vi "COVIDxPLORE.vi"() -> ()   [LabVIEW 2017]
panel:
  in  "LeftTab":enum32{"Page 1", "Page 2"}(tab)
  out "How many days until zero growth?":string
  out "Is there a trend in the growth?":string
  out "Is the infection growing?":string
  out "What part of the population is infected?":string
  out "How many are infected?":string
  out "How many days until zero growth?":string
  out "Is there a trend in the growth of dead?":string
  out "Are the number of dead growing?":string
  out "What part of the population has died?":string
  out "How many are dead?":string
  in  "RightTabs":enum32{"Plots", "GeoSelect"}(tab)
  in  "Fixed":T1
  in  "Days":i32
  in  "ZoomToDays":bool
  in  "ResetGraph":bool
  in  "GotoGeo":bool
  in  "Plots":u16(ring) items=["Modoc County Dead", "Modoc County Infected", "Siskiyou County Dead", "Siskiyou County Infected", "Humboldt County Dead", "Humboldt County Infected", "Washoe County Dead", "Washoe County Infected", "Benton County Dead", "Benton County Infected", "Crook County Dead", "Crook County Infected", "Deschutes County Dead", "Deschutes County Infected", "Douglas County Dead", "Douglas County Infected", "Grant County Dead", "Grant County Infected", "Harney County Dead", "Harney County Infected", "Jackson County Dead", "Jackson County Infected", "Jefferson County Dead", "Jefferson County Infected", "Klamath County Dead", "Klamath County Infected", "Lake County Dead", "Lake County Infected", "Lane County Dead", "Lane County Infected", "Lincoln County Dead", "Lincoln County Infected", "Linn County Dead", "Linn County Infected", "Marion County Dead", "Marion County Infected", "Wasco County Dead", "Wasco County Infected", "Combined Dead", "Combined Infected"]
  out "Plot":cluster{"Days":timestamp[], dbl[]}[](graph)
  in  "GotoPlots":bool
  in  "Clear":bool
  in  "Level":u16(ring) items=["County", "State", "Country"]
  in  "Expand":bool
  in  "Add":bool
  out "Days of data":i32
  out "Last day of data":timestamp format="%<%m/%d>T"
  out "Regions":string[][](table)
  in  "Lookup":bool
  in  "Find by":u16(ring) items=["Zipcode", "CountyName", "StateName", "CountyFips", "StateFips", "StateAbbr", "CityState"]
  in  "GeoData":T2
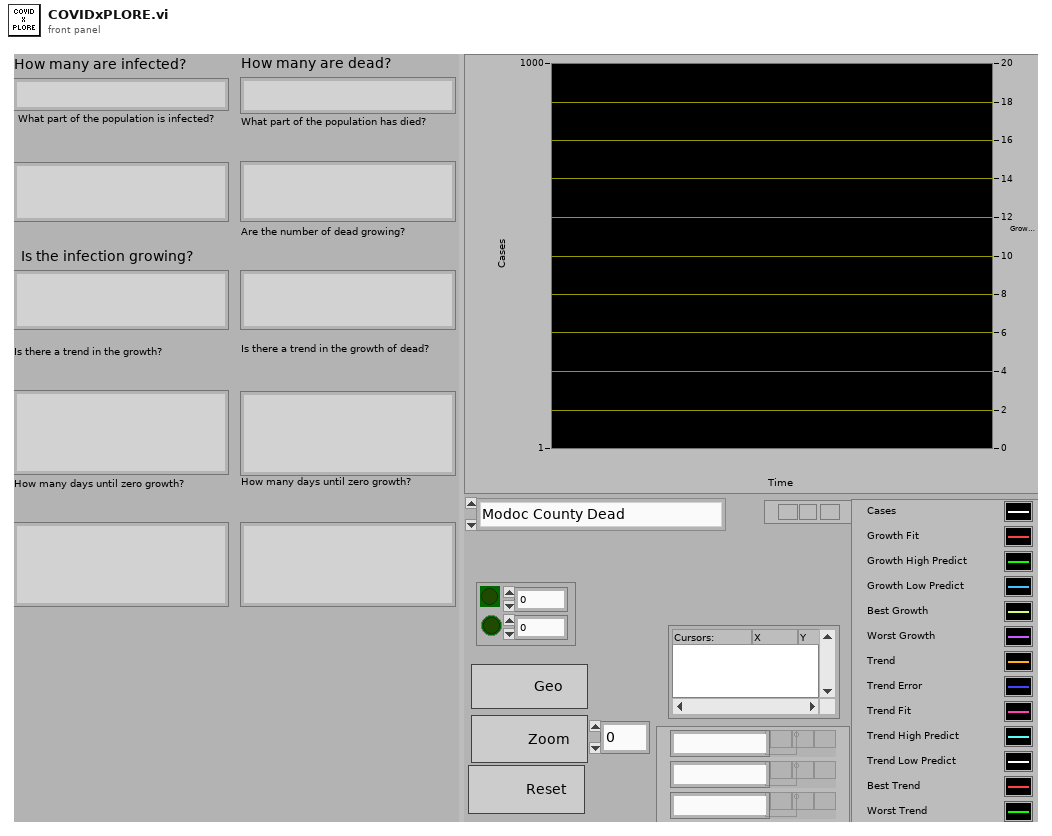
[diagram p1: front panel]
types:
  T1 = cluster{"FixedGrowth":bool, "DaysBackGrowth":dbl, "FixedTrend":bool, "DaysBackTrend":dbl}
  T2 = cluster{"Zip":i32, "CountyFIPS":i32, "StateFips":i32, "CountyName":string, "StateName":string, "StateAbbr":string, "City":string}
  T3 = enum16{"LoadData", "GetStateData", "GetCountyData", "GetCountyArray"}
  T4 = enum16{"ClearCache", "AddPlot", "GetPlot", "GetNames", "LastPlot"}
  T5 = enum16{"Zipcode", "CountyName", "StateName", "CountyFips", "StateFips", "StateAbbr", "CityState"}
  T6 = enum16{"AddEntry", "Clear", "Expand", "Combine", "GetStrings"}
  T7 = enum16{"AddEntry", "Clear", "Expand", "Combine", "GetStrings", "GetGeo"}
  T8 = cluster{"Infected":string, "InfectedRate":string, "InfectionGrowth":string, "GrowthTrend":string, "DaysToZero":string, "Dead":string, "CFR":string, "CFR Growth":string, "CFRtrend":string, "DaysToZeroDead":string}
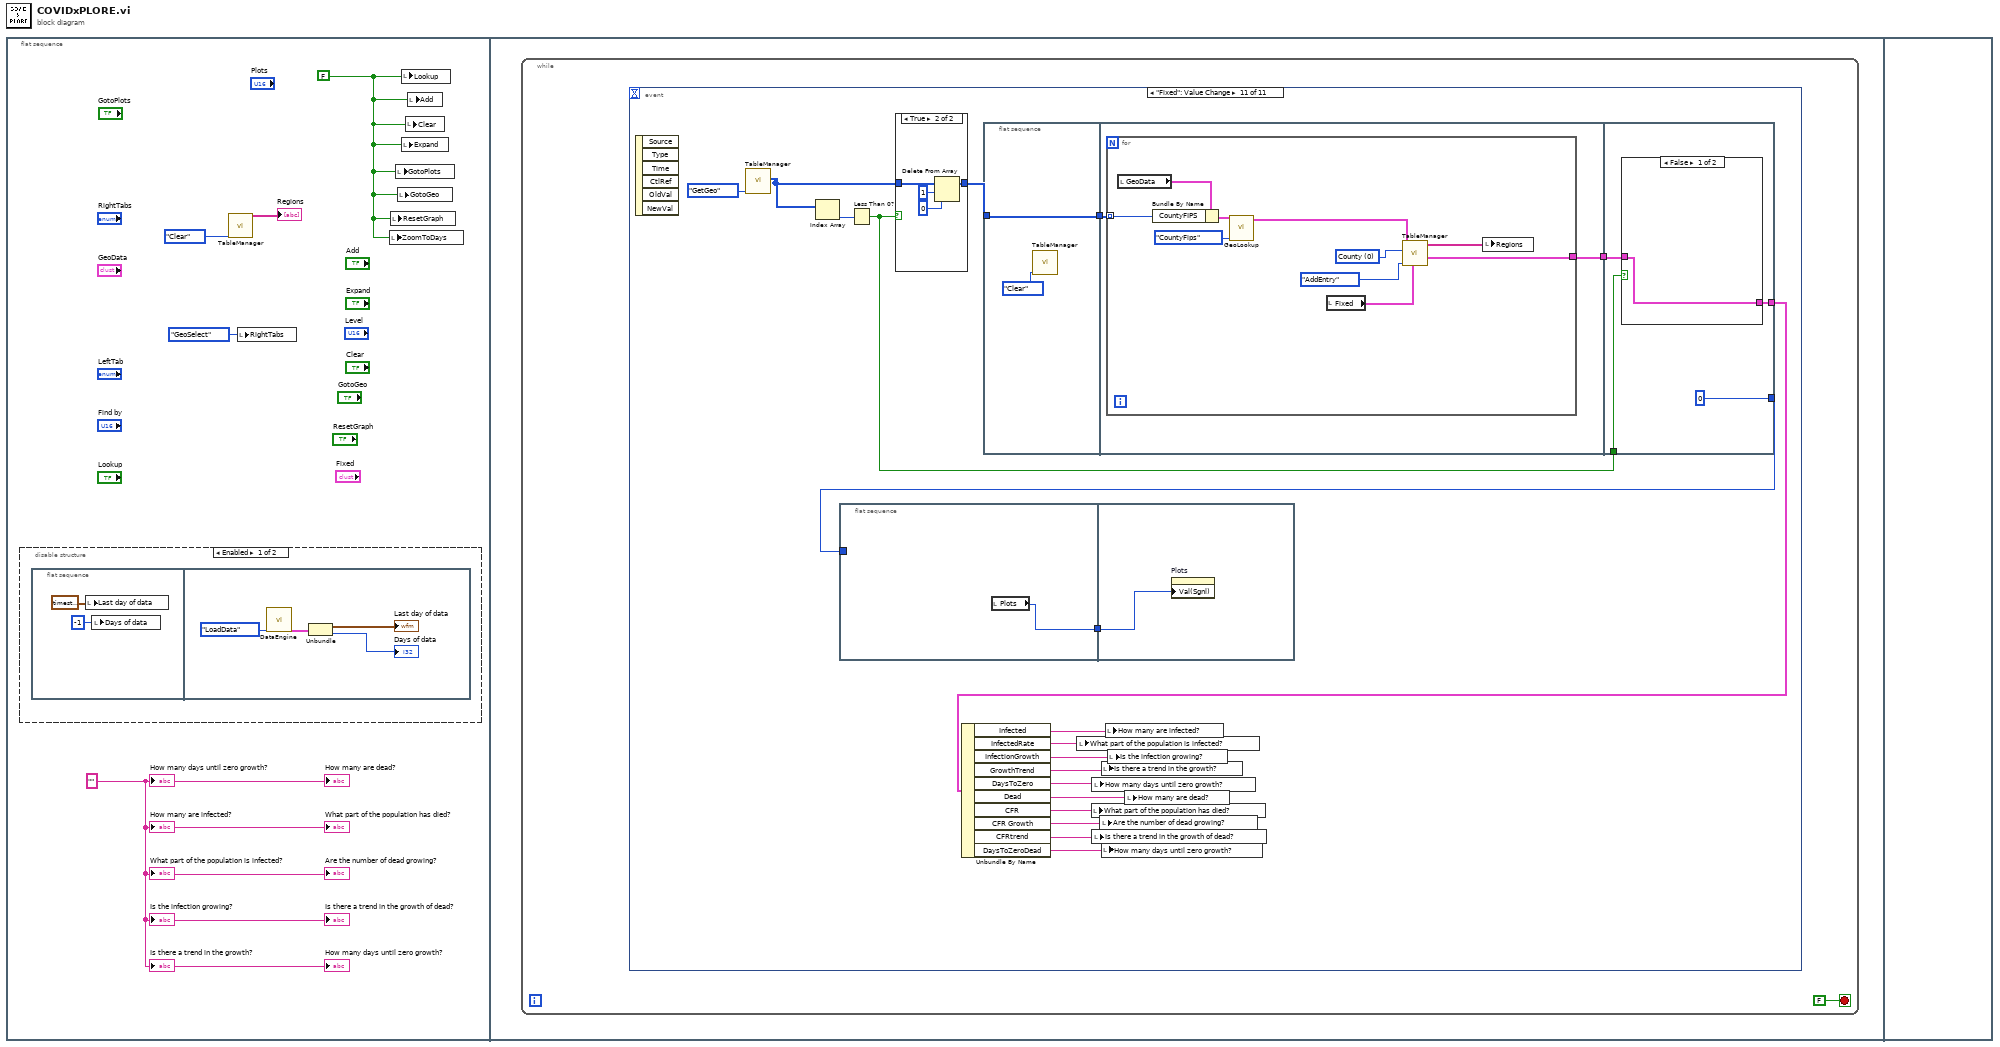
[diagram p0: block diagram]
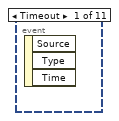
[diagram p3: hidden frame]
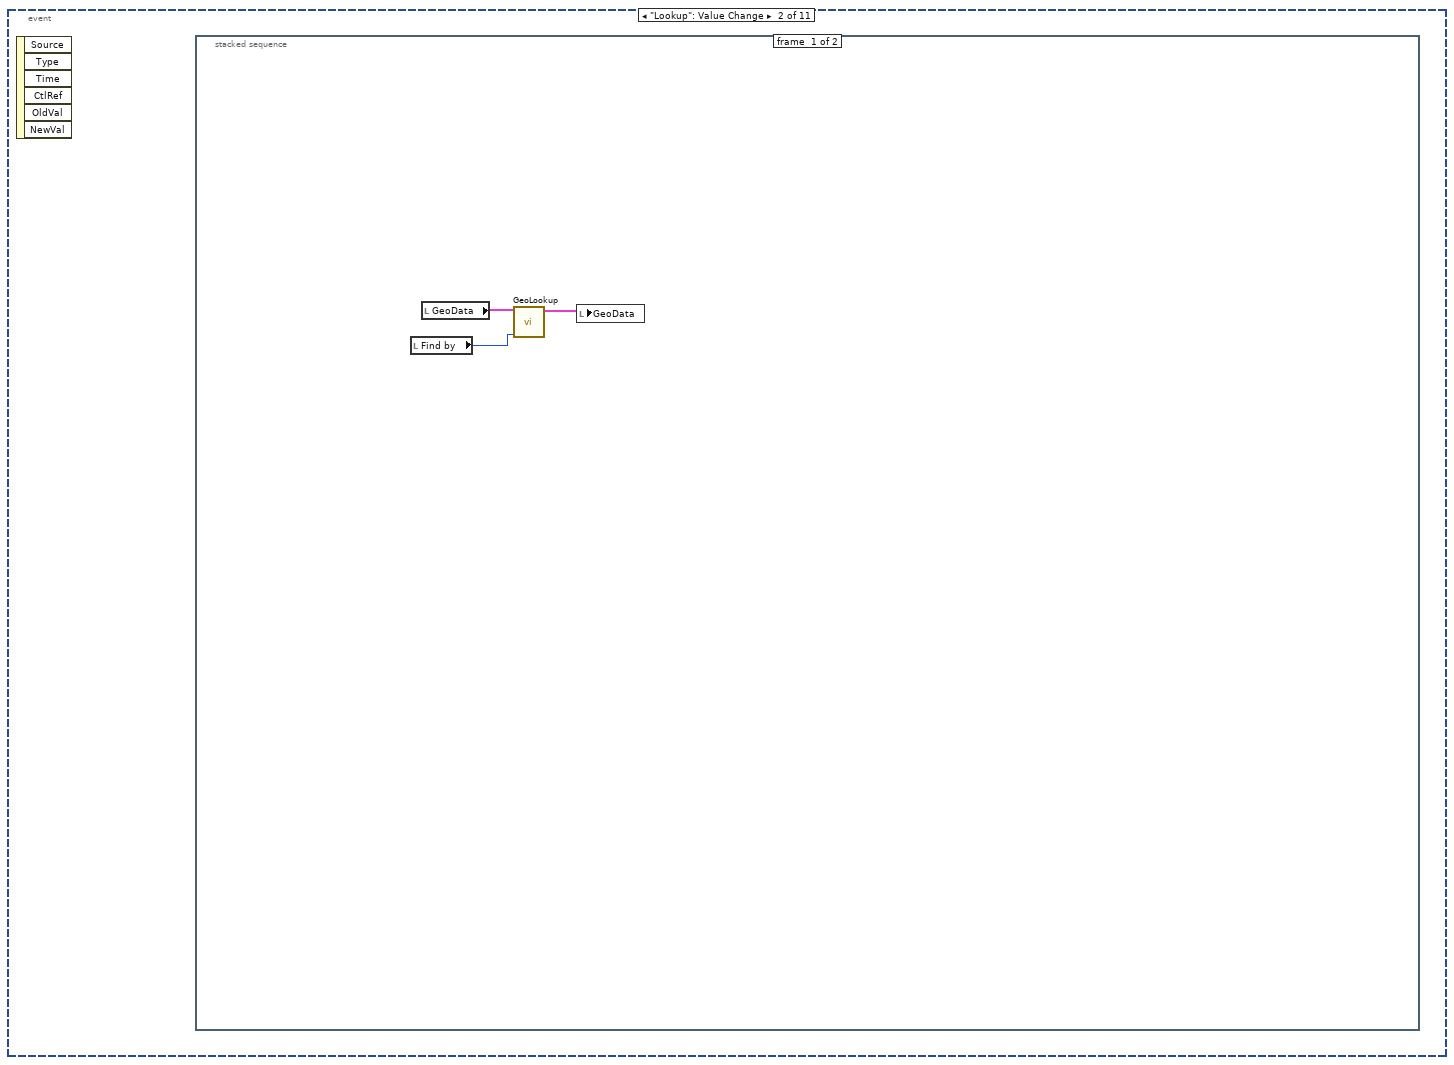
[diagram p4: hidden frame]
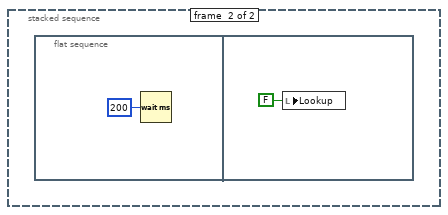
[diagram p5: hidden frame]
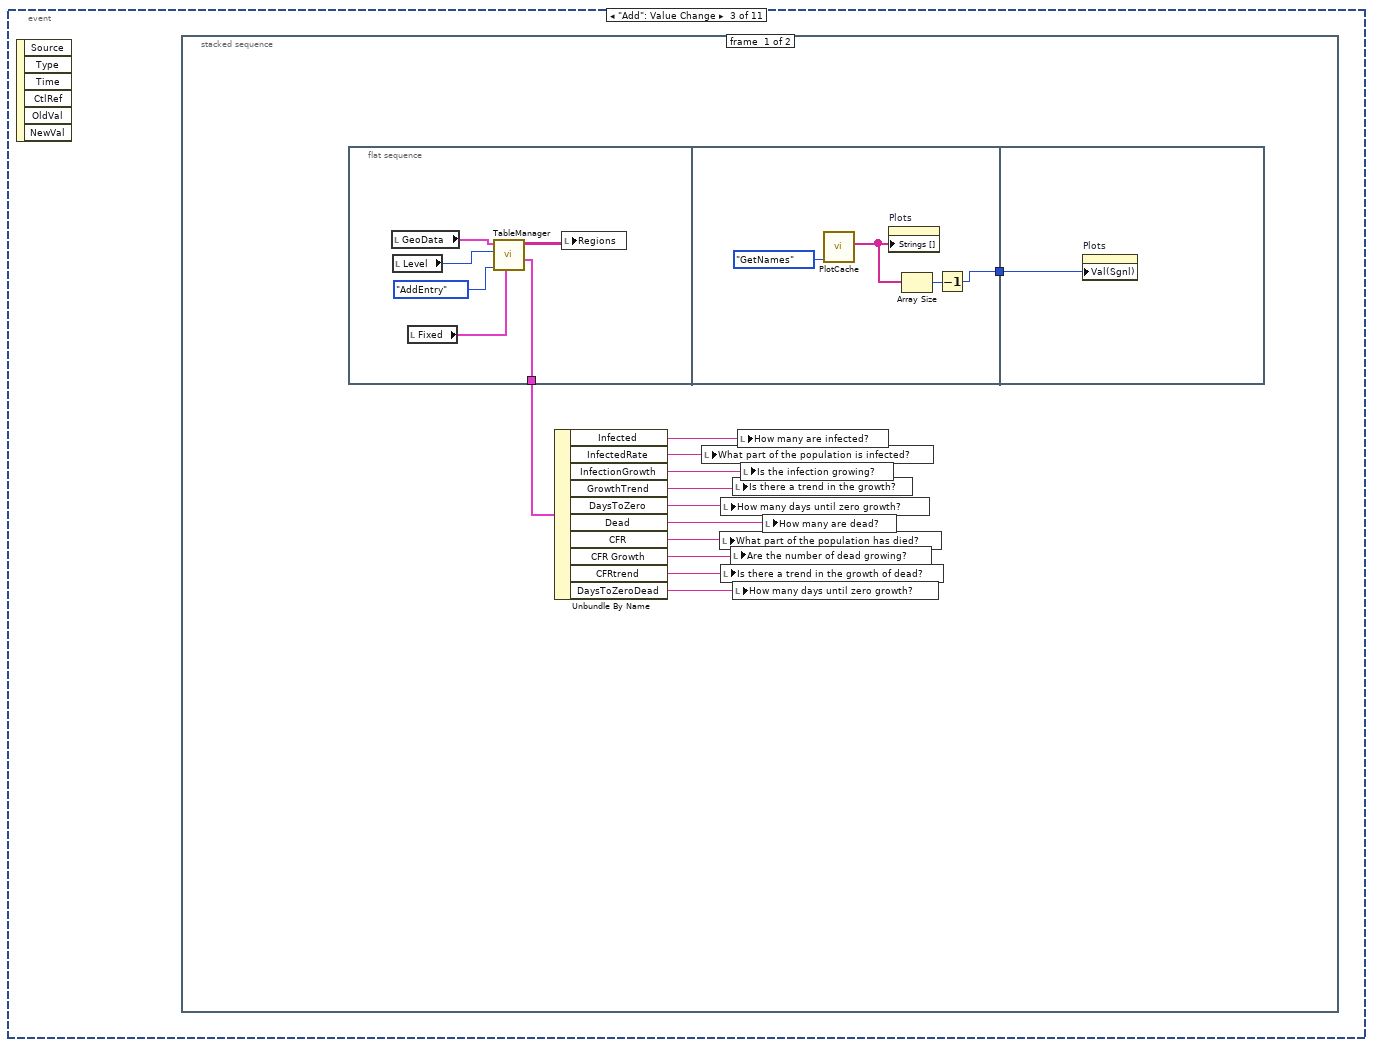
[diagram p6: hidden frame]
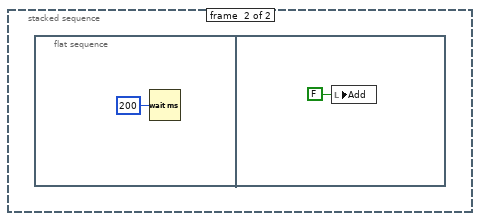
[diagram p7: hidden frame]
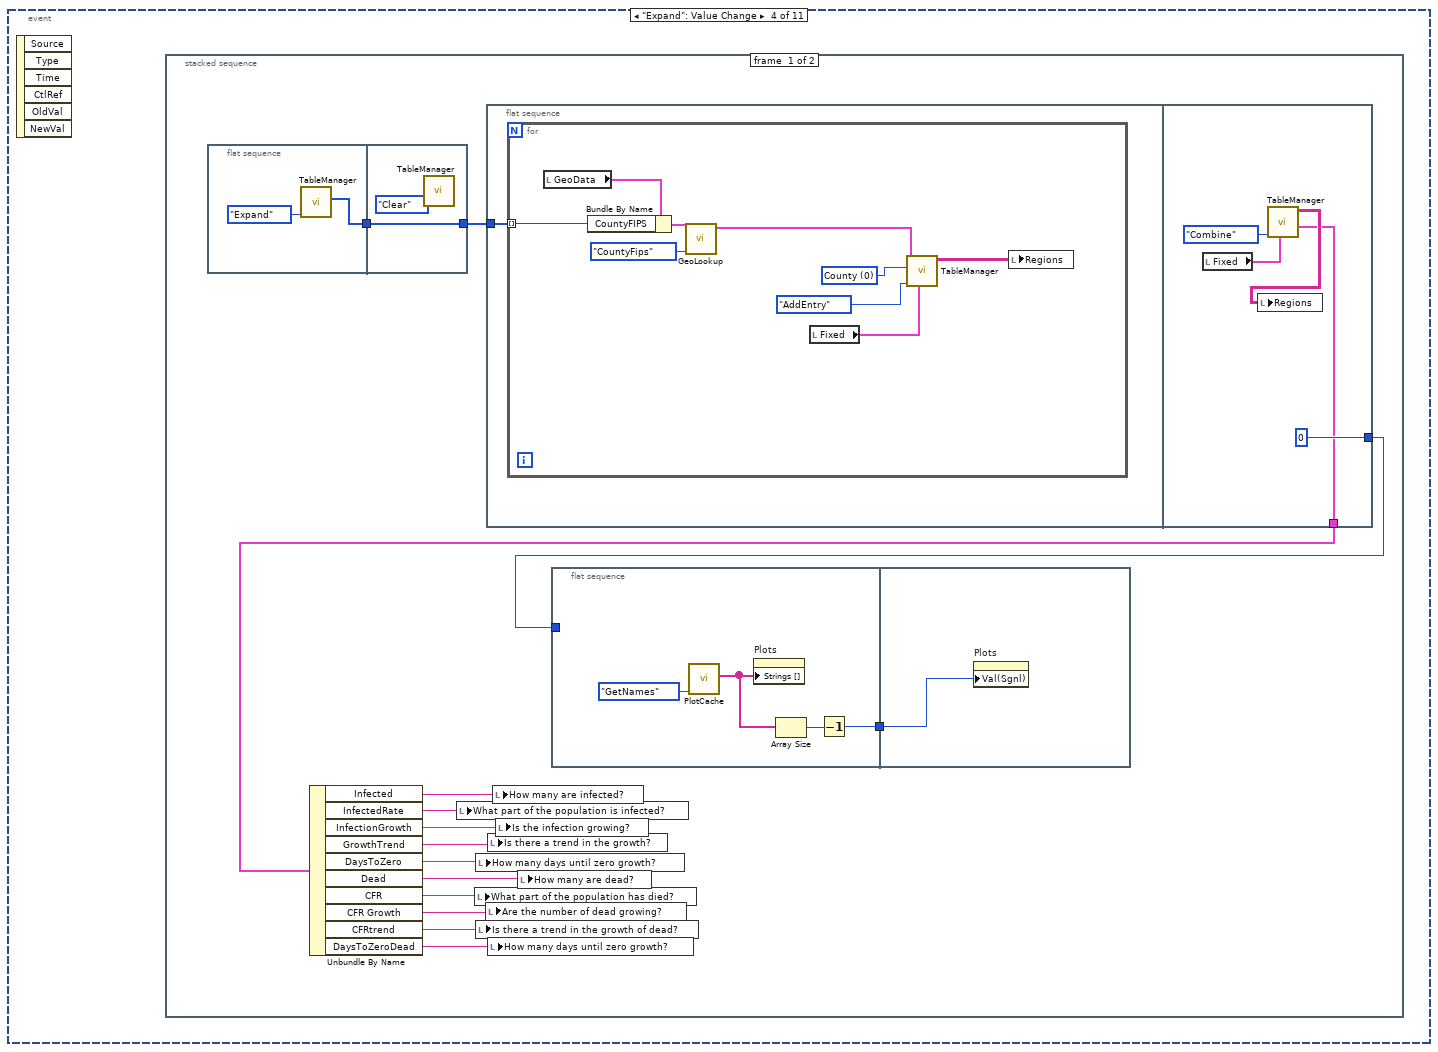
[diagram p8: hidden frame]
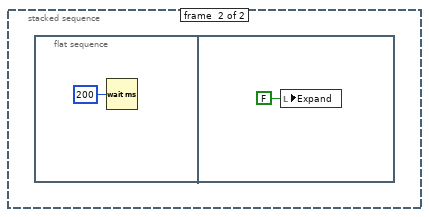
[diagram p9: hidden frame]
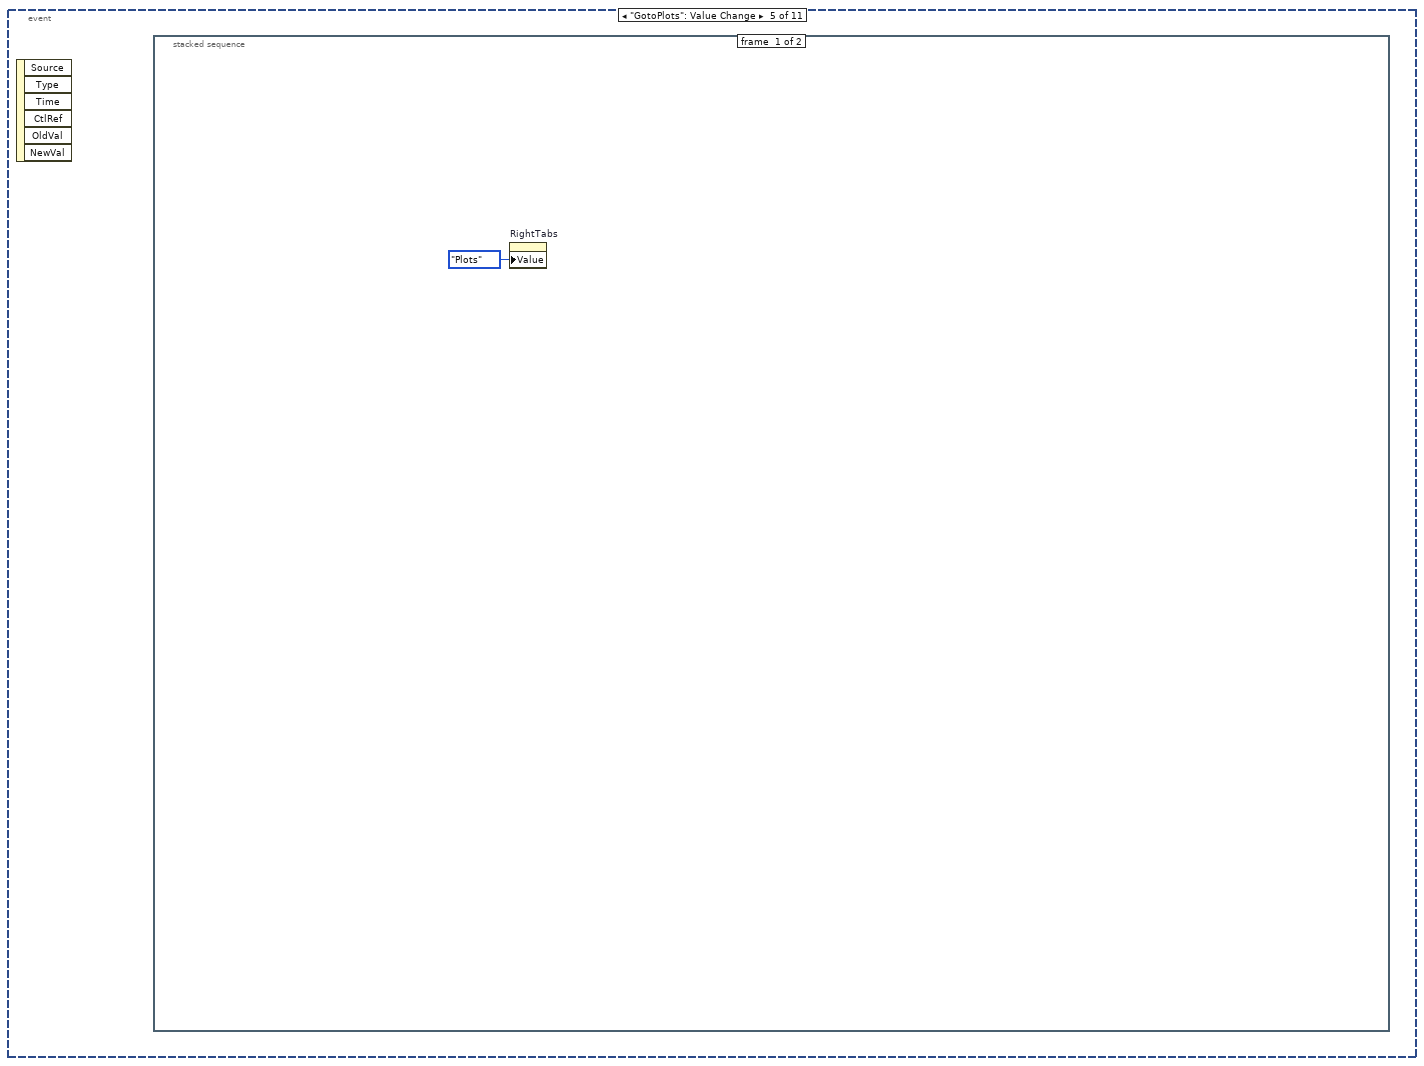
[diagram p10: hidden frame]
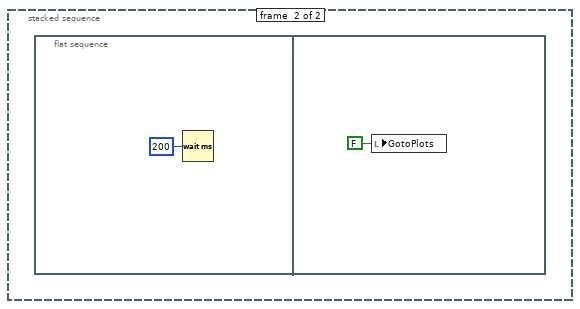
[diagram p11: hidden frame]
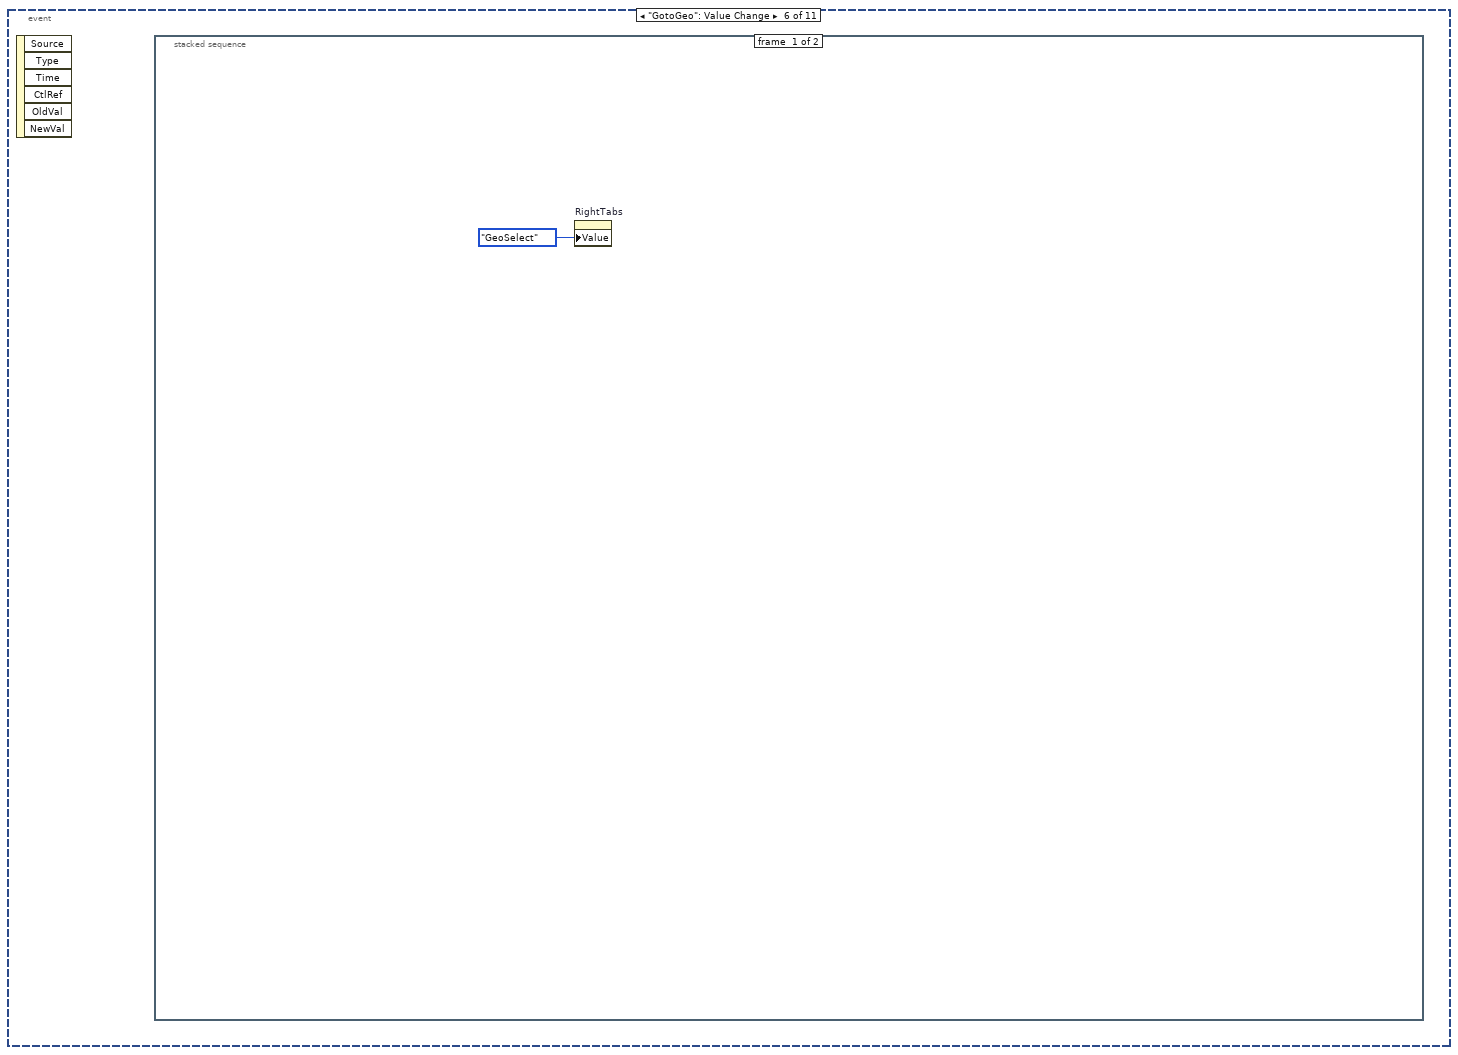
[diagram p12: hidden frame]
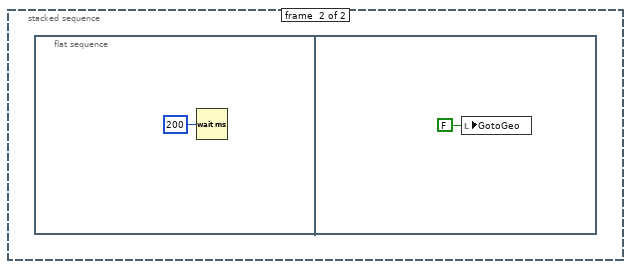
[diagram p13: hidden frame]
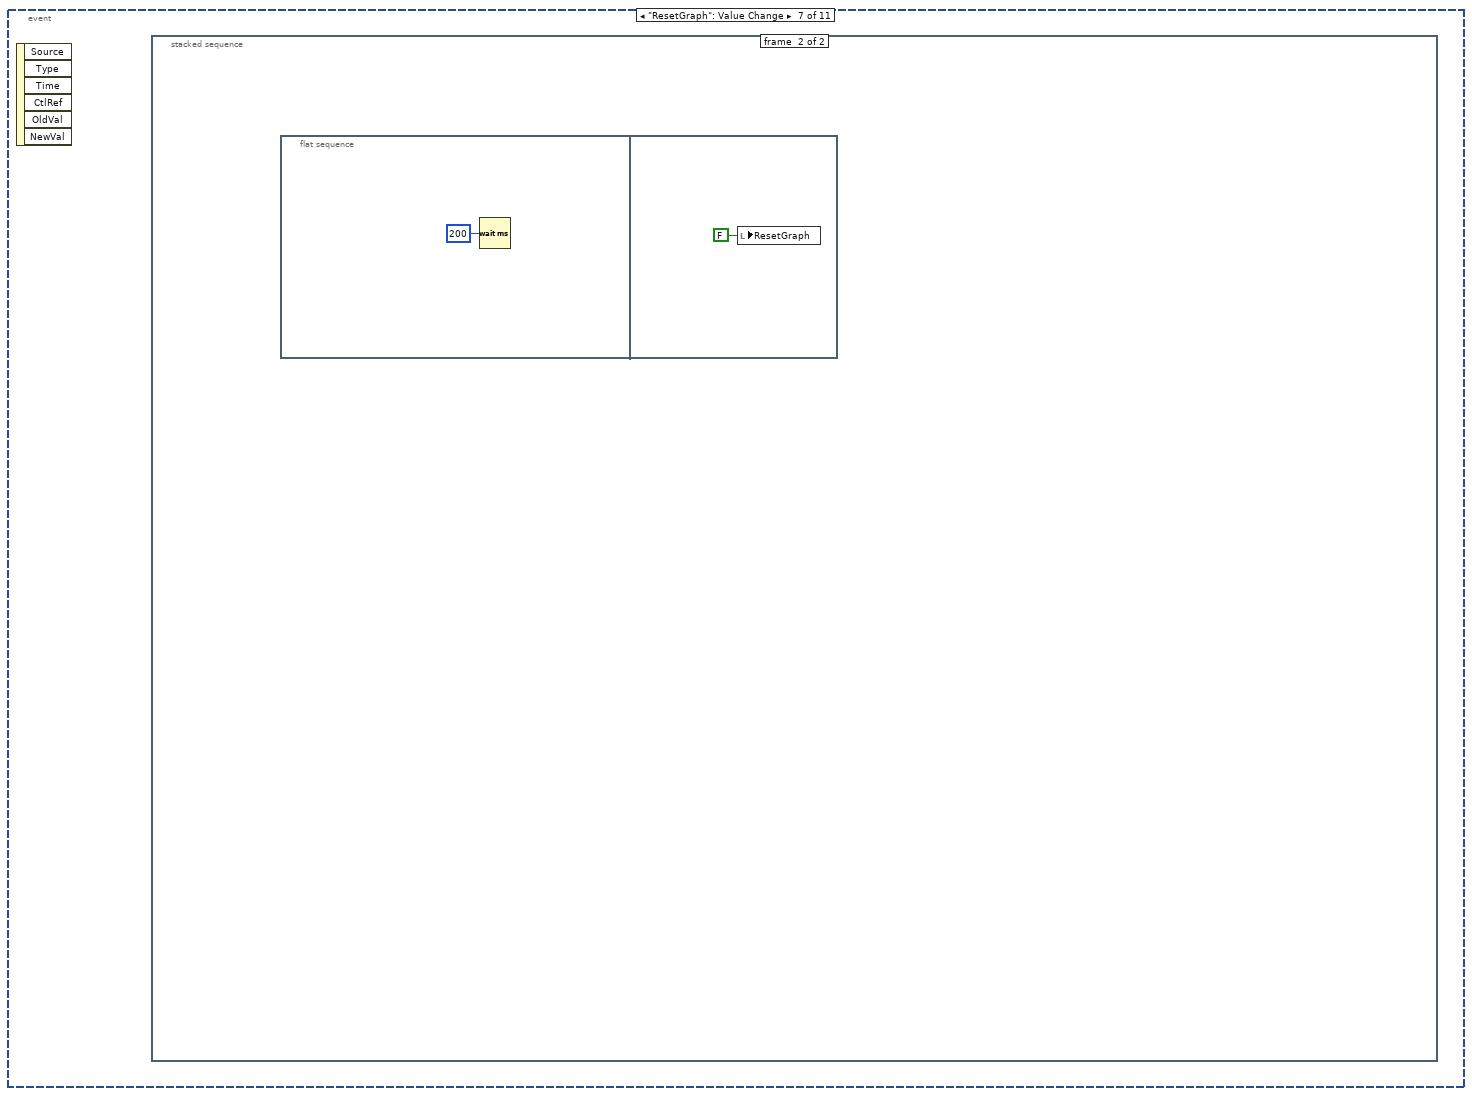
[diagram p14: hidden frame]
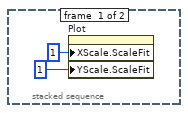
[diagram p15: hidden frame]
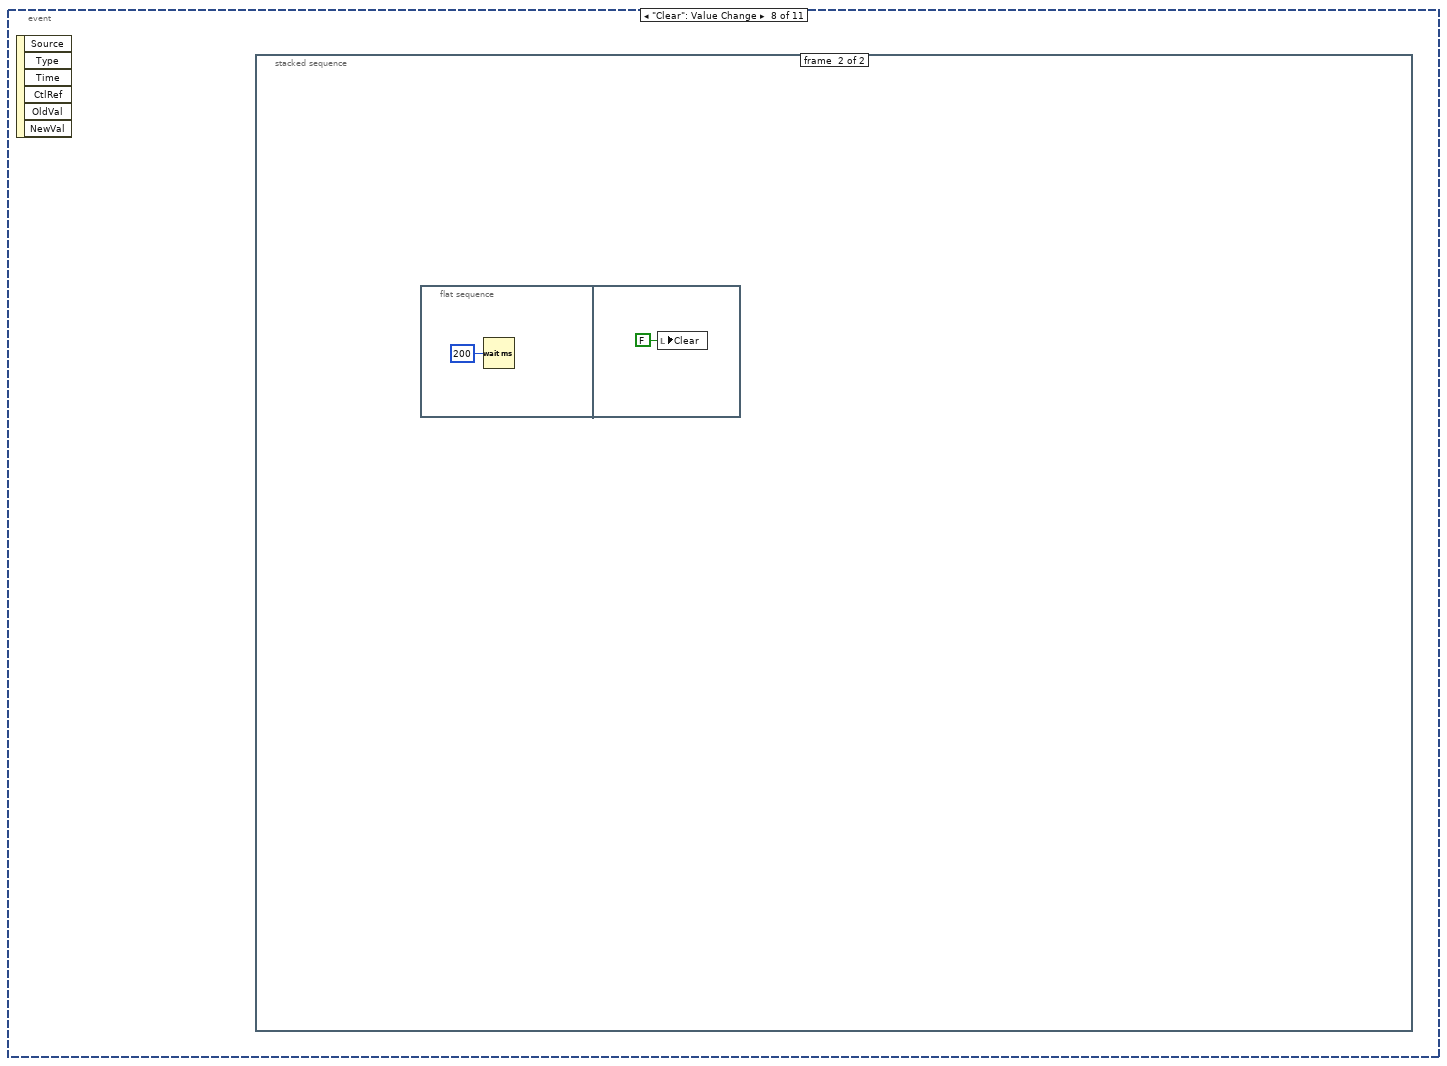
[diagram p16: hidden frame]
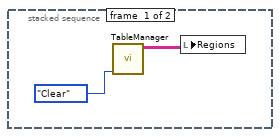
[diagram p17: hidden frame]
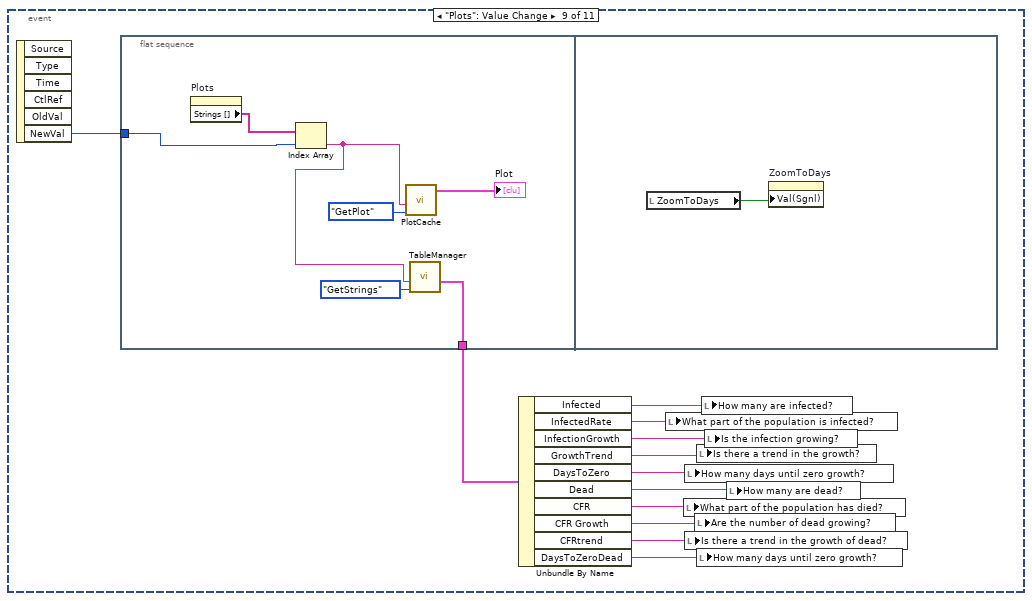
[diagram p18: hidden frame]
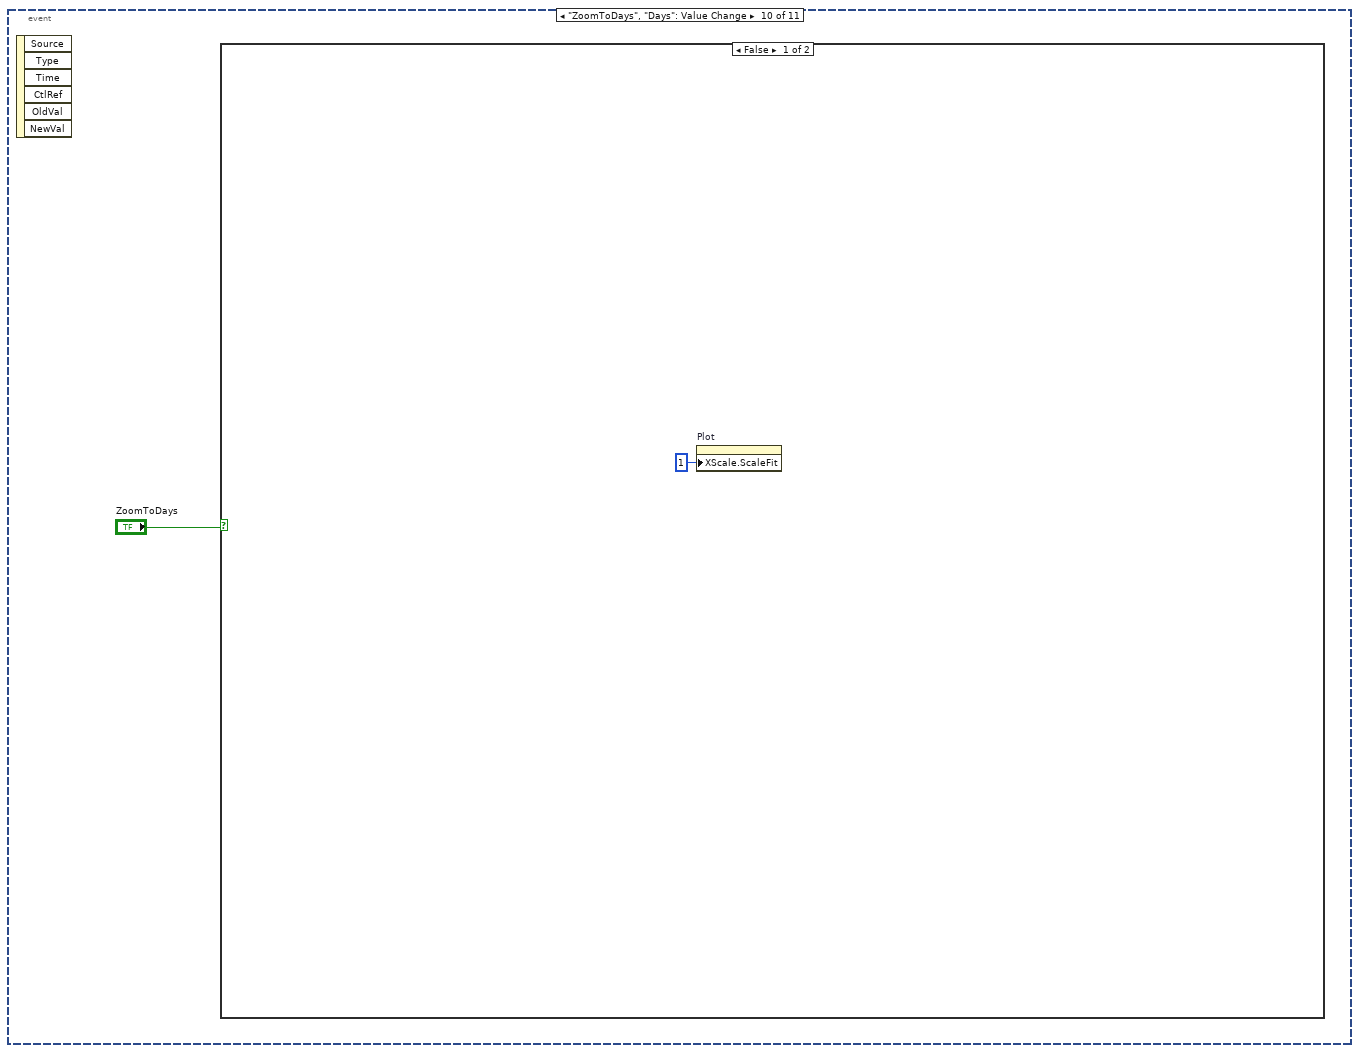
[diagram p19: hidden frame]
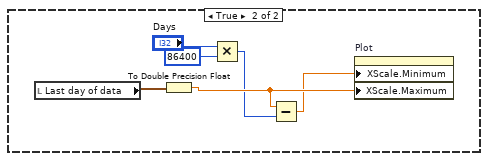
[diagram p20: hidden frame]
diagram:
  n1 = flat-sequence {
    frame #0 {
      w3 = ""
      w2 = FALSE ("Lookup")
      n2 = disable-structure shown="Enabled" {
        frame Enabled {
          n3 = flat-sequence {
            frame #0 {
              n4 = local write "Last day of data"(timestamp(3691731600 s since 1904-01-01) ("Last day of data")) -> ()
              n5 = local write "Days of data"(-1 ("Days of data")) -> ()
            }
            frame #1 {
              n6 = call "DataEngine.vi"("Op"=T3."LoadData") -> ("UpdateInfo"=w10:cluster{"time stamp":timestamp, i32})  [unwired: 9 in, 1 out]
              n7 = Unbundle(w10) -> ("time stamp"=→"Last day of data":timestamp, →"Days of data":i32)
            }
          }
        }
        frame Disabled {
        }
      }
      n8 = call "TableManager.vi"("Op"=enum16{"AddEntry", "Clear", "Expand"}."Clear") -> ("TableOut"=→"Regions":string[][])  [unwired: 8 in, 2 out]
      n9 = local write "RightTabs"(enum32{"Plots", "GeoSelect"}."GeoSelect" ("RightTabs")) -> ()
      n10 = local write "ZoomToDays"(w2) -> ()
      n11 = local write "ResetGraph"(w2) -> ()
      n12 = local write "GotoPlots"(w2) -> ()
      n13 = local write "GotoGeo"(w2) -> ()
      n14 = local write "Lookup"(w2) -> ()
      n15 = local write "Expand"(w2) -> ()
      n16 = local write "Clear"(w2) -> ()
      n17 = local write "Add"(w2) -> ()
      "How many are infected?" <- w3
      "What part of the population is infected?" <- w3
      "Is the infection growing?" <- w3
      "Is there a trend in the growth?" <- w3
      "How many days until zero growth?" <- w3
      "How many are dead?" <- w3
      "What part of the population has died?" <- w3
      "Are the number of dead growing?" <- w3
      "Is there a trend in the growth of dead?" <- w3
      "How many days until zero growth?" <- w3
    }
    frame #1 {
      n18 = while {
        stop <- FALSE stop-if-true
        n19 = event shown="[10] \"Fixed\": Value Change" {
          selector: _ -> [_ _ _ _ _ _ _ _ _ _ _]
          dyn-events: _ -> [_ _ _ _ _ _ _ _ _ _ _]
          timeout: _ -> [_ _ _ _ _ _ _ _ _ _ _]
          event Timeout {
            n20 = event-data() -> ()  [unwired: 1 in, 3 out]
          }
          event "Lookup": Value Change {
            n21 = event-data() -> ()  [unwired: 1 in, 6 out]
            n22 = stacked-sequence {
              frame #0 {
                n23 = local read "Find by"() -> (w14:u16)
                n24 = local read "GeoData"() -> (w15:T2)
                n25 = call "GeoLookup.vi"("Type"=w14, "Data"=w15) -> ("DataOut"=w13:T2)  [unwired: 9 in]
                n26 = local write "GeoData"(w13) -> ()
              }
              frame #1 {
                n27 = flat-sequence {
                  frame #0 {
                    n28 = Wait (ms)(milliseconds to wait=u32 200) -> ()  [unwired: 1 out]
                  }
                  frame #1 {
                    n29 = local write "Lookup"(FALSE ("Lookup")) -> ()
                  }
                }
              }
            }
          }
          event "Add": Value Change {
            n30 = event-data() -> ()  [unwired: 1 in, 6 out]
            n31 = stacked-sequence {
              frame #0 {
                n32 = flat-sequence {
                  tunnel: [w31] -> w28
                  tunnel: [w36] -> w29
                  tunnel: w29 -> [w40]
                  frame #0 {
                    n33 = local read "GeoData"() -> (w35:T2)
                    n34 = local read "Level"() -> (w34:u16)
                    n35 = local read "Fixed"() -> (w30:T1)
                    n36 = call "TableManager.vi"("Fixed"=w30, "Op"=enum16{"AddEntry", "Clear"}."AddEntry", "Level"=w34, "GeoData"=w35) -> ("Strings"=w31:T8, "TableOut"=w32:string[][])  [unwired: 5 in, 1 out]
                    n37 = local write "Regions"(w32) -> ()
                  }
                  frame #1 {
                    n38 = call "PlotCache.vi"("Op"=T4."GetNames") -> ("Names"=w38:string[])  [unwired: 8 in, 2 out]
                    n39 = property on="Plots" class="Ring (strict)"("Strings []"=w38) -> ()  [unwired: 2 in, 2 out]
                    n40 = Array Size(array=w38) -> (size(s)=w37:i32)
                    n41 = Decrement(x=w37) -> (x-1=w36:i32)
                  }
                  frame #2 {
                    n42 = property on="Plots" class="Ring (strict)"("Val(Sgnl)"=w40) -> ()  [unwired: 2 in, 2 out]
                  }
                }
                n43 = Unbundle By Name(w28) -> ("Infected"=w27:string, "InfectedRate"=w26:string, "InfectionGrowth"=w25:string, "GrowthTrend"=w24:string, "DaysToZero"=w23:string, "Dead"=w22:string, "CFR"=w21:string, "CFR Growth"=w20:string, "CFRtrend"=w19:string, "DaysToZeroDead"=w18:string)
                n44 = local write "What part of the population is infected?"(w26) -> ()
                n45 = local write "What part of the population has died?"(w21) -> ()
                n46 = local write "How many days until zero growth?"(w23) -> ()
                n47 = local write "Is there a trend in the growth of dead?"(w19) -> ()
                n48 = local write "Are the number of dead growing?"(w20) -> ()
                n49 = local write "Is there a trend in the growth?"(w24) -> ()
                n50 = local write "How many days until zero growth?"(w18) -> ()
                n51 = local write "How many are infected?"(w27) -> ()
                n52 = local write "Is the infection growing?"(w25) -> ()
                n53 = local write "How many are dead?"(w22) -> ()
              }
              frame #1 {
                n54 = flat-sequence {
                  frame #0 {
                    n55 = Wait (ms)(milliseconds to wait=u32 200) -> ()  [unwired: 1 out]
                  }
                  frame #1 {
                    n56 = local write "Add"(FALSE ("Add")) -> ()
                  }
                }
              }
            }
          }
          event "Expand": Value Change {
            n57 = event-data() -> ()  [unwired: 1 in, 6 out]
            n58 = stacked-sequence {
              frame #0 {
                n59 = flat-sequence {
                  tunnel: [w78] -> w56
                  tunnel: [w80] -> w57
                  tunnel: w56 -> [w80]
                  frame #0 {
                    n60 = call "TableManager.vi"("Op"=enum16{"AddEntry", "Clear", "Expand"}."Expand") -> ("FipsOut"=w78:i32[])  [unwired: 8 in, 2 out]
                  }
                  frame #1 {
                    n61 = call "TableManager.vi"("Op"=enum16{"AddEntry", "Clear", "Expand"}."Clear") -> ()  [unwired: 8 in, 3 out]
                  }
                }
                n62 = Unbundle By Name(w43) -> ("Infected"=w53:string, "InfectedRate"=w52:string, "InfectionGrowth"=w51:string, "GrowthTrend"=w50:string, "DaysToZero"=w49:string, "Dead"=w48:string, "CFR"=w47:string, "CFR Growth"=w46:string, "CFRtrend"=w45:string, "DaysToZeroDead"=w44:string)
                n63 = local write "What part of the population is infected?"(w52) -> ()
                n64 = local write "What part of the population has died?"(w47) -> ()
                n65 = local write "How many days until zero growth?"(w49) -> ()
                n66 = local write "Is there a trend in the growth of dead?"(w45) -> ()
                n67 = local write "Are the number of dead growing?"(w46) -> ()
                n68 = flat-sequence {
                  tunnel: w57 -> [w63]
                  tunnel: [0] -> w55
                  tunnel: [w74] -> w43
                  frame #0 {
                    n69 = for {
                      tunnel: w63 -> [w71] mode=indexing
                      w66 = u16 0 items=["County", "State", "Country"] ("Level")
                      n70 = local read "GeoData"() -> (w72:T2)
                      n71 = Bundle By Name(cluster=w72, "CountyFIPS"=w71) -> (w70:T2)
                      n72 = call "GeoLookup.vi"("Type"=T5."CountyFips", "Data"=w70) -> ("DataOut"=w65:T2)  [unwired: 9 in]
                      n73 = local read "Fixed"() -> (w64:T1)
                      n74 = call "TableManager.vi"("Fixed"=w64, "Op"=enum16{"AddEntry", "Clear", "Expand"}."AddEntry", "Level"=w66, "GeoData"=w65) -> ("TableOut"=w68:string[][])  [unwired: 5 in, 2 out]
                      n75 = local write "Regions"(w68) -> ()
                    }
                  }
                  frame #1 {
                    n76 = local read "Fixed"() -> (w73:T1)
                    n77 = call "TableManager.vi"("Fixed"=w73, "Op"=enum16{"AddEntry", "Clear", "Expand", "Combine"}."Combine") -> ("Strings"=w74:T8, "TableOut"=w76:string[][])  [unwired: 7 in, 1 out]
                    n78 = local write "Regions"(w76) -> ()
                  }
                }
                n79 = local write "Is there a trend in the growth?"(w50) -> ()
                n80 = local write "How many days until zero growth?"(w44) -> ()
                n81 = local write "How many are infected?"(w53) -> ()
                n82 = local write "Is the infection growing?"(w51) -> ()
                n83 = local write "How many are dead?"(w48) -> ()
                n84 = flat-sequence {
                  tunnel: w55 -> [_]
                  tunnel: [w58] -> w54
                  tunnel: w54 -> [w62]
                  frame #0 {
                    n85 = call "PlotCache.vi"("Op"=T4."GetNames") -> ("Names"=w60:string[])  [unwired: 8 in, 2 out]
                    n86 = property on="Plots" class="Ring (strict)"("Strings []"=w60) -> ()  [unwired: 2 in, 2 out]
                    n87 = Array Size(array=w60) -> (size(s)=w59:i32)
                    n88 = Decrement(x=w59) -> (x-1=w58:i32)
                  }
                  frame #1 {
                    n89 = property on="Plots" class="Ring (strict)"("Val(Sgnl)"=w62) -> ()  [unwired: 2 in, 2 out]
                  }
                }
              }
              frame #1 {
                n90 = flat-sequence {
                  frame #0 {
                    n91 = Wait (ms)(milliseconds to wait=u32 200) -> ()  [unwired: 1 out]
                  }
                  frame #1 {
                    n92 = local write "Expand"(FALSE ("Expand")) -> ()
                  }
                }
              }
            }
          }
          event "GotoPlots": Value Change {
            n93 = event-data() -> ()  [unwired: 1 in, 6 out]
            n94 = stacked-sequence {
              frame #0 {
                n95 = property on="RightTabs" class="TabCtl (strict)"("Value"=enum32{"Plots", "GeoSelect"}."Plots" ("RightTabs")) -> ()  [unwired: 2 in, 2 out]
              }
              frame #1 {
                n96 = flat-sequence {
                  frame #0 {
                    n97 = Wait (ms)(milliseconds to wait=u32 200) -> ()  [unwired: 1 out]
                  }
                  frame #1 {
                    n98 = local write "GotoPlots"(FALSE ("GotoPlots")) -> ()
                  }
                }
              }
            }
          }
          event "GotoGeo": Value Change {
            n99 = event-data() -> ()  [unwired: 1 in, 6 out]
            n100 = stacked-sequence {
              frame #0 {
                n101 = property on="RightTabs" class="TabCtl (strict)"("Value"=enum32{"Plots", "GeoSelect"}."GeoSelect" ("Value (Signaling)")) -> ()  [unwired: 2 in, 2 out]
              }
              frame #1 {
                n102 = flat-sequence {
                  frame #0 {
                    n103 = Wait (ms)(milliseconds to wait=u32 200) -> ()  [unwired: 1 out]
                  }
                  frame #1 {
                    n104 = local write "GotoGeo"(FALSE ("GotoGeo")) -> ()
                  }
                }
              }
            }
          }
          event "ResetGraph": Value Change {
            n105 = event-data() -> ()  [unwired: 1 in, 6 out]
            n106 = stacked-sequence {
              frame #0 {
                n107 = property on="Plot" class="XYGraph (strict)"("XScale.ScaleFit"=u8 1 ("X Scale.Scale Fit"), "YScale.ScaleFit"=u8 1 ("Y Scale.Scale Fit")) -> ()  [unwired: 2 in, 2 out]
              }
              frame #1 {
                n108 = flat-sequence {
                  frame #0 {
                    n109 = Wait (ms)(milliseconds to wait=u32 200) -> ()  [unwired: 1 out]
                  }
                  frame #1 {
                    n110 = local write "ResetGraph"(FALSE ("ResetGraph")) -> ()
                  }
                }
              }
            }
          }
          event "Clear": Value Change {
            n111 = event-data() -> ()  [unwired: 1 in, 6 out]
            n112 = stacked-sequence {
              frame #0 {
                n113 = call "TableManager.vi"("Op"=enum16{"AddEntry", "Clear"}."Clear") -> ("TableOut"=w94:string[][])  [unwired: 8 in, 2 out]
                n114 = local write "Regions"(w94) -> ()
              }
              frame #1 {
                n115 = flat-sequence {
                  frame #0 {
                    n116 = Wait (ms)(milliseconds to wait=u32 200) -> ()  [unwired: 1 out]
                  }
                  frame #1 {
                    n117 = local write "Clear"(FALSE ("Add")) -> ()
                  }
                }
              }
            }
          }
          event "Plots": Value Change {
            n118 = event-data() -> ("NewVal"=w109:u16)  [unwired: 1 in, 5 out]
            n119 = flat-sequence {
              tunnel: w109 -> [w112]
              tunnel: [w111] -> w98
              frame #0 {
                n120 = property on="Plots" class="Ring (strict)"() -> ("Strings []"=w115:string[])  [unwired: 2 in, 2 out]
                n121 = Index Array(array=w115, index=w112) -> (element=w110:string)
                n122 = call "PlotCache.vi"("Op"=T4."GetPlot", "PlotName"=w110) -> ("PlotOut"=→"Plot":cluster{"Days":timestamp[], dbl[]}[])  [unwired: 7 in, 2 out]
                n123 = call "TableManager.vi"("Op"=T6."GetStrings", "PlotName"=w110) -> ("Strings"=w111:T8)  [unwired: 7 in, 2 out]
              }
              frame #1 {
                n124 = local read "ZoomToDays"() -> (w117:bool)
                n125 = property on="ZoomToDays" class="Bool (strict)"("Val(Sgnl)"=w117) -> ()  [unwired: 2 in, 2 out]
              }
            }
            n126 = Unbundle By Name(w98) -> ("Infected"=w108:string, "InfectedRate"=w107:string, "InfectionGrowth"=w106:string, "GrowthTrend"=w105:string, "DaysToZero"=w104:string, "Dead"=w103:string, "CFR"=w102:string, "CFR Growth"=w101:string, "CFRtrend"=w100:string, "DaysToZeroDead"=w99:string)
            n127 = local write "What part of the population is infected?"(w107) -> ()
            n128 = local write "What part of the population has died?"(w102) -> ()
            n129 = local write "How many days until zero growth?"(w104) -> ()
            n130 = local write "Is there a trend in the growth of dead?"(w100) -> ()
            n131 = local write "Are the number of dead growing?"(w101) -> ()
            n132 = local write "Is there a trend in the growth?"(w105) -> ()
            n133 = local write "How many days until zero growth?"(w99) -> ()
            n134 = local write "How many are infected?"(w108) -> ()
            n135 = local write "Is the infection growing?"(w106) -> ()
            n136 = local write "How many are dead?"(w103) -> ()
          }
          event "ZoomToDays", "Days": Value Change {
            n137 = event-data() -> ()  [unwired: 1 in, 6 out]
            n138 = case shown="False" "ZoomToDays" {
              frame False {
                n139 = property on="Plot" class="XYGraph (strict)"("XScale.ScaleFit"=u8 1 ("X Scale.Scale Fit")) -> ()  [unwired: 2 in, 2 out]
              }
              frame True {
                n140 = local read "Last day of data"() -> (w125:timestamp)
                n141 = To Double Precision Float(number=w125) -> (double precision float=w124:dbl)
                n142 = Multiply(x="Days", y=86400) -> (x*y=w121:i32)
                n143 = Subtract(x=w124, y=w121) -> (x-y=w120:dbl)
                n144 = property on="Plot" class="XYGraph (strict)"("XScale.Minimum"=w120, "XScale.Maximum"=w124) -> ()  [unwired: 2 in, 2 out]
              }
            }
          }
          event "Fixed": Value Change {
            n145 = event-data() -> ()  [unwired: 1 in, 6 out]
            n146 = call "TableManager.vi"("Op"=T7."GetGeo") -> ("FipsOut"=w143:i32[])  [unwired: 8 in, 2 out]
            n147 = Index Array(array=w143) -> (element=w144:i32)  [unwired: 1 in]
            n148 = flat-sequence {
              tunnel: w139 -> [_]
              tunnel: [w146] -> w140
              tunnel: w140 -> [w147]
              frame #0 {
                n149 = local read "Plots"() -> (w146:u16)
              }
              frame #1 {
                n150 = property on="Plots" class="Ring (strict)"("Val(Sgnl)"=w147) -> ()  [unwired: 2 in, 2 out]
              }
            }
            n151 = Less Than 0?(x=w144) -> (x < 0?=w141:bool)
            n152 = case shown="True" w141 {
              tunnel: w143 -> [w171 w175]
              tunnel: [w171 w172] -> w142
              frame False {
              }
              frame True {
                n153 = Delete From Array(array=w175, length=1, index=0) -> (array with subset deleted=w172:i32[])  [unwired: 1 out]
              }
            }
            n154 = Unbundle By Name(w128) -> ("Infected"=w138:string, "InfectedRate"=w137:string, "InfectionGrowth"=w136:string, "GrowthTrend"=w135:string, "DaysToZero"=w134:string, "Dead"=w133:string, "CFR"=w132:string, "CFR Growth"=w131:string, "CFRtrend"=w130:string, "DaysToZeroDead"=w129:string)
            n155 = flat-sequence {
              tunnel: w142 -> [w149]
              tunnel: [w149] -> w126
              tunnel: [w150] -> w127
              tunnel: w126 -> [w151]
              tunnel: w141 -> [w165]
              tunnel: [0] -> w139
              tunnel: [w163] -> w128
              tunnel: w127 -> [w162]
              frame #0 {
                n156 = call "TableManager.vi"("Op"=T7."Clear") -> ()  [unwired: 8 in, 3 out]
              }
              frame #1 {
                n157 = for {
                  tunnel: w151 -> [w160] mode=indexing
                  tunnel: [w152] -> w150
                  w155 = u16 0 items=["County", "State", "Country"] ("Level")
                  n158 = local read "GeoData"() -> (w161:T2)
                  n159 = Bundle By Name(cluster=w161, "CountyFIPS"=w160) -> (w159:T2)
                  n160 = call "GeoLookup.vi"("Type"=T5."CountyFips", "Data"=w159) -> ("DataOut"=w154:T2)  [unwired: 9 in]
                  n161 = local read "Fixed"() -> (w153:T1)
                  n162 = call "TableManager.vi"("Fixed"=w153, "Op"=enum16{"AddEntry", "Clear", "Expand"}."AddEntry", "Level"=w155, "GeoData"=w154) -> ("Strings"=w152:T8, "TableOut"=w157:string[][])  [unwired: 5 in, 1 out]
                  n163 = local write "Regions"(w157) -> ()
                }
              }
              frame #2 {
                n164 = case shown="False" w165 {
                  tunnel: [w166 w167] -> w163
                  tunnel: w162 -> [w166 w167]
                  frame False {
                  }
                  frame True {
                    n165 = local read "Fixed"() -> (w168:T1)
                    n166 = call "TableManager.vi"("Fixed"=w168, "Op"=enum16{"AddEntry", "Clear", "Expand", "Combine"}."Combine") -> ("TableOut"=w169:string[][])  [unwired: 7 in, 2 out]
                    n167 = local write "Regions"(w169) -> ()
                  }
                }
              }
            }
            n168 = local write "What part of the population is infected?"(w137) -> ()
            n169 = local write "What part of the population has died?"(w132) -> ()
            n170 = local write "How many days until zero growth?"(w134) -> ()
            n171 = local write "Is there a trend in the growth of dead?"(w130) -> ()
            n172 = local write "Are the number of dead growing?"(w131) -> ()
            n173 = local write "Is there a trend in the growth?"(w135) -> ()
            n174 = local write "How many days until zero growth?"(w129) -> ()
            n175 = local write "How many are infected?"(w138) -> ()
            n176 = local write "Is the infection growing?"(w136) -> ()
            n177 = local write "How many are dead?"(w133) -> ()
          }
        }
      }
    }
    frame #2 {
    }
  }
